vi "TestSetOutWave.vi"(8 "error in (no error)":errorcluster) -> (0 "error out":errorcluster)   [LabVIEW 2020]
uses:
  <vilib>/addons/_JKI Toolkits/Caraya/classes/Test/Test.lvclass
  <vilib>/addons/_JKI Toolkits/Caraya/classes/Assert/Assert.lvclass
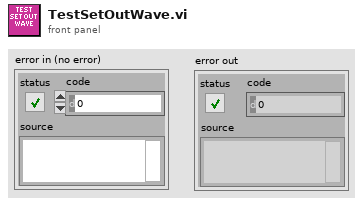
[diagram p1: front panel]
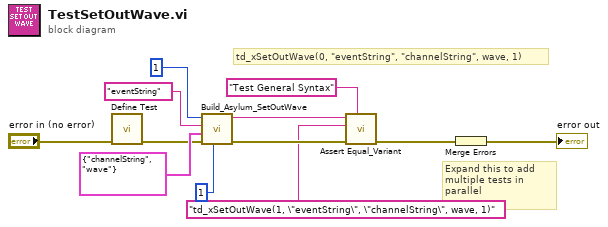
[diagram p0: block diagram]
diagram:
  # "td_xSetOutWave(0, \"eventString\", \"channelString\", wave, 1)"
  # "Expand this to add multiple tests in parallel"
  n1 = call <vilib>:"Define Test.vi"("error in (no error)"="error in (no error)") -> ("error out"=w4:errorcluster)  [unwired: 10 in]
  n2 = call "Build_Asylum_SetOutWave.vi"("interpolation"=1, "error in (no error)"=w4, "Wave"=cluster{"channelString":string, "wave":string} {"channelString"="channelString", "wave"="wave"}, "eventString"="eventString", "whichBank"=1) -> ("error out"=w2:errorcluster, "Command"=w3:string)  [unwired: 5 in]
  n3 = call <vilib>:"Assert Equal_Variant.vi"("Label"="Test General Syntax", "error in (no error)"=w2, "Y"="td_xSetOutWave(1, \"eventString\", \"channelString\", wave, 1)", "X"=w3) -> ("error out"=w10:errorcluster)  [unwired: 7 in]
  n4 = Merge Errors(w10) -> (→"error out":errorcluster)
